vi "运维调试_采配水.vi"() -> ()   [LabVIEW 2016, in "PLC.lvlib"]
uses:
  PLC.lvlib
  <vilib>/Plasmionique/MB Master/MB_Master/MB_Master.lvclass
  <vilib>/Utility/miscctls.llb/LVPointTypeDef.ctl
  <vilib>/Plasmionique/MB Master/MB_Master_Serial/MB_Master_Serial.lvclass
  D:/Program Files (x86)/National Instruments/LabVIEW 2016/vi.lib/Plasmionique/MB Master/MB_Master/MB_Master.lvclass
  <vilib>/Utility/config.llb/Read Key (U32).vi
  <vilib>/Plasmionique/MB Master/MB Master.lvlib
  <vilib>/Utility/config.llb/NI_LVConfig.lvlib
panel:
  out "R22":i16
  in  "V8":bool
  out "R111":i16 caption="排液时间"
  out "通讯故障":bool
  out "R21":i16
  in  "V7":bool
  out "R20":i16
  in  "M1-2":bool
  in  "潜水泵工作模式":u16(ring) items=["泵1单泵单管路", "泵2单泵单管路", "双泵双管路"]
  out "X10":bool caption="废液报警"
  out "X9":bool caption="自来水报警"
  out "X8":bool caption="泵2过载报警"
  out "X7":bool caption="泵1过载报警"
  out "X6":bool caption="断电检测"
  out "X5":bool caption="开门检测"
  out "X4":bool caption="烟雾检测"
  out "X3":bool caption="漏水检测"
  out "X2":bool caption="进样检测"
  out "X1":bool
  out "X0":bool caption="采样池液位开关"
  out "Y12":bool caption="多参通电"
  out "R109":i16 caption="配水时间"
  out "集成报警信息":string
  out "R108":i16 caption="自来水报警"
  out "R107":i16 caption="采水池液位报警设置"
  out "R106":i16 caption="进样超时设置"
  out "R105":i16 caption="二级清洗时间"
  out "R104":i16 caption="一级清洗时间"
  out "R103":i16 caption="外部管路清洗时间"
  out "R102":i16 caption="静置沉淀时间"
  out "R101":i16 caption="内部管路润洗时间"
  out "R100":i16 caption="外部管路润洗时间"
  out "R2":i16
  out "R1":i16
  out "多列列表框":i32(listbox)
  out "R19":i16
  in  "V6":bool
  out "R18":i16
  in  "V5":bool
  out "R17":i16
  in  "V4":bool
  out "R16":i16
  in  "V3":bool
  out "R15":i16
  in  "V2":bool
  out "R14":i16
  in  "M2":bool
  out "R13":i16
  in  "V1":bool
  out "R12":i16
  in  "M1-1":bool
  in  "返回":bool
  in  "参数设置":bool
  in  "单步启动":bool
  in  "启动":bool
  in  "停止":bool
  # "S"
  # "S"
  # "S"
  # "S"
  # "S"
  # "S"
  # "S"
  # "S"
  # "S"
  # "S"
  # "S"
  # "单步计时："
  # "s"
  # "流程计时："
  # "s"
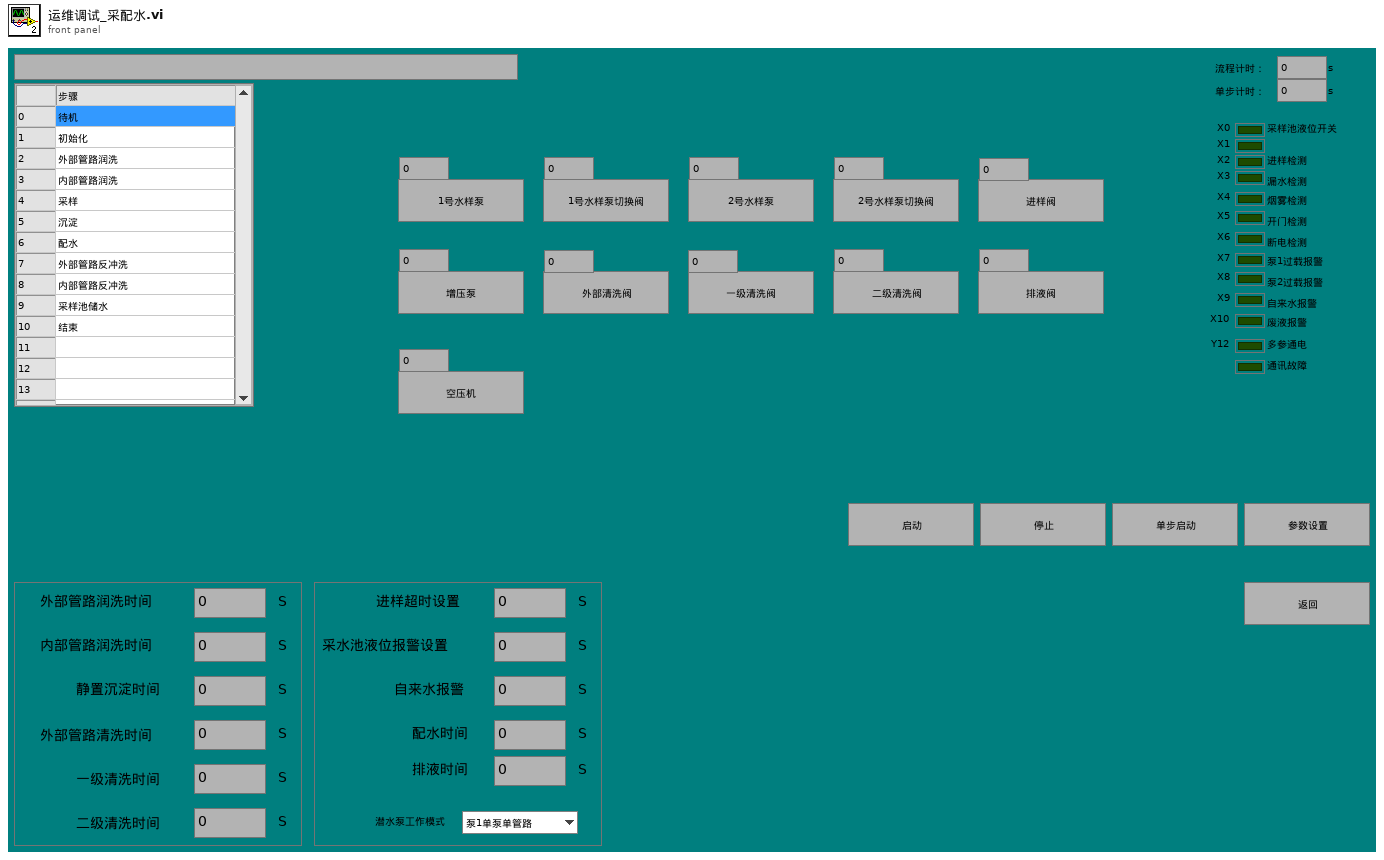
[diagram p1: front panel]
types:
  T1 = typedef "LVPointTypeDef.ctl" = cluster{"Horizontal":i16, "Vertical":i16}
  T2 = cluster{"时间标识":timestamp, "设备":string, "日志信息":string}
  T3 = cluster{"R0":i16, "R1":i16, "R2":i16, "R3":i16, "R4":i16, "R5":i16, "R6":i16, "R7":i16, "R8":i16, "R9":i16, "R10":i16, "R11":i16, "R12":i16, "R13":i16, "R14":i16, "R15":i16, "R16":i16, "R17":i16, "R18":i16, "R19":i16, "R20":i16, "R21":i16, "R22":i16}
  T4 = cluster{"coil values[0]":bool, "coil values[1]":bool, "coil values[2]":bool, "coil values[3]":bool, "coil values[4]":bool, "coil values[5]":bool, "coil values[6]":bool, "coil values[7]":bool, "coil values[8]":bool, "coil values[9]":bool, "coil values[10]":bool, "coil values[11]":bool, "coil values[12]":bool, "coil values[13]":bool, "coil values[14]":bool, "coil values[15]":bool}
  T5 = cluster{"seconds since 1Jan1904":timestamp, "table输入":string, string, "table输入":string}
  T6 = cluster{"时间标识":timestamp, "设备":string, "日志信息":string, "流程参数":string}
  T7 = cluster{"命令":string, cluster{"starting address":u16, "holding register value":u16}}
  T8 = cluster{"是否启用仪器":bool, "CODMn":cluster{"启动测量模式":cluster{"测量模式":enum16{"水样测量", "标样核查", "零点核查", "加标回收", "平行样", "校零", "校标"}}, "确定按钮":bool}, "采水模式":enum16{"使用采水泵", "不使用采水泵"}}
  T9 = enum16{"水样测量", "标样核查", "零点核查", "加标回收", "平行样", "校零", "校标"}
  T10 = cluster{"命令":string, "数据":cluster{"starting address":u16, "holding register value":u16}}
  T11 = cluster{"命令":string, "数据":cluster{"starting address":u16, "holding register values":u16[]}}
  T12 = cluster{"命令":string, "data":cluster{"starting address":u16, "coil values":bool[]}}
  T13 = enum32{"Bad", "Idle", "Run top level", "Running"}
  T14 = typedef "NI_LVConfig.lvlib/Config Data RefNum.ctl" = refnum<k1>
  T15 = cluster{"baud rate (bps)":u32, "stop bits":u16, "parity":u16, "flow control":u16, "timeout":u32, "retries":i32}
  T16 = cluster{"starting address":u16, "holding register values":u16[]}
  T17 = cluster{"starting address":u16, "holding register value":u16}
  T18 = cluster{"starting address":u16, "coil values":bool[]}
  T19 = cluster{"Registers[0]":u16, "Registers[1]":u16, "Registers[2]":u16, "Registers[3]":u16, "Registers[4]":u16, "Registers[5]":u16, "Registers[6]":u16, "Registers[7]":u16, "Registers[8]":u16, "Registers[9]":u16, "Registers[10]":u16, "Registers[11]":u16, "Registers[12]":u16, "Registers[13]":u16, "Registers[14]":u16, "Registers[15]":u16, "Registers[16]":u16, "Registers[17]":u16, "Registers[18]":u16, "Registers[19]":u16, "Registers[20]":u16, "Registers[21]":u16, "Registers[22]":u16}
  T20 = cluster{"Registers[0]":u16, "Registers[1]":u16, "Registers[2]":u16, "Registers[3]":u16, "Registers[4]":u16, "Registers[5]":u16}
  T21 = cluster{"Coils[0]":bool, "Coils[1]":bool, "Coils[2]":bool, "Coils[3]":bool, "Coils[4]":bool, "Coils[5]":bool, "Coils[6]":bool, "Coils[7]":bool, "Coils[8]":bool, "Coils[9]":bool, "Coils[10]":bool, "Coils[11]":bool, "Coils[12]":bool, "Coils[13]":bool, "Coils[14]":bool, "Coils[15]":bool}
  T22 = cluster{"Registers[0]":u16, "Registers[1]":u16, "Registers[2]":u16, "Registers[3]":u16, "Registers[4]":u16, "Registers[5]":u16, "Registers[6]":u16, "Registers[7]":u16, "Registers[8]":u16, "Registers[9]":u16, "Registers[10]":u16, "Registers[11]":u16, "Registers[12]":u16, "Registers[13]":u16, "Registers[14]":u16, "Registers[15]":u16, "Registers[16]":u16, "Registers[17]":u16, "Registers[18]":u16, "Registers[19]":u16}
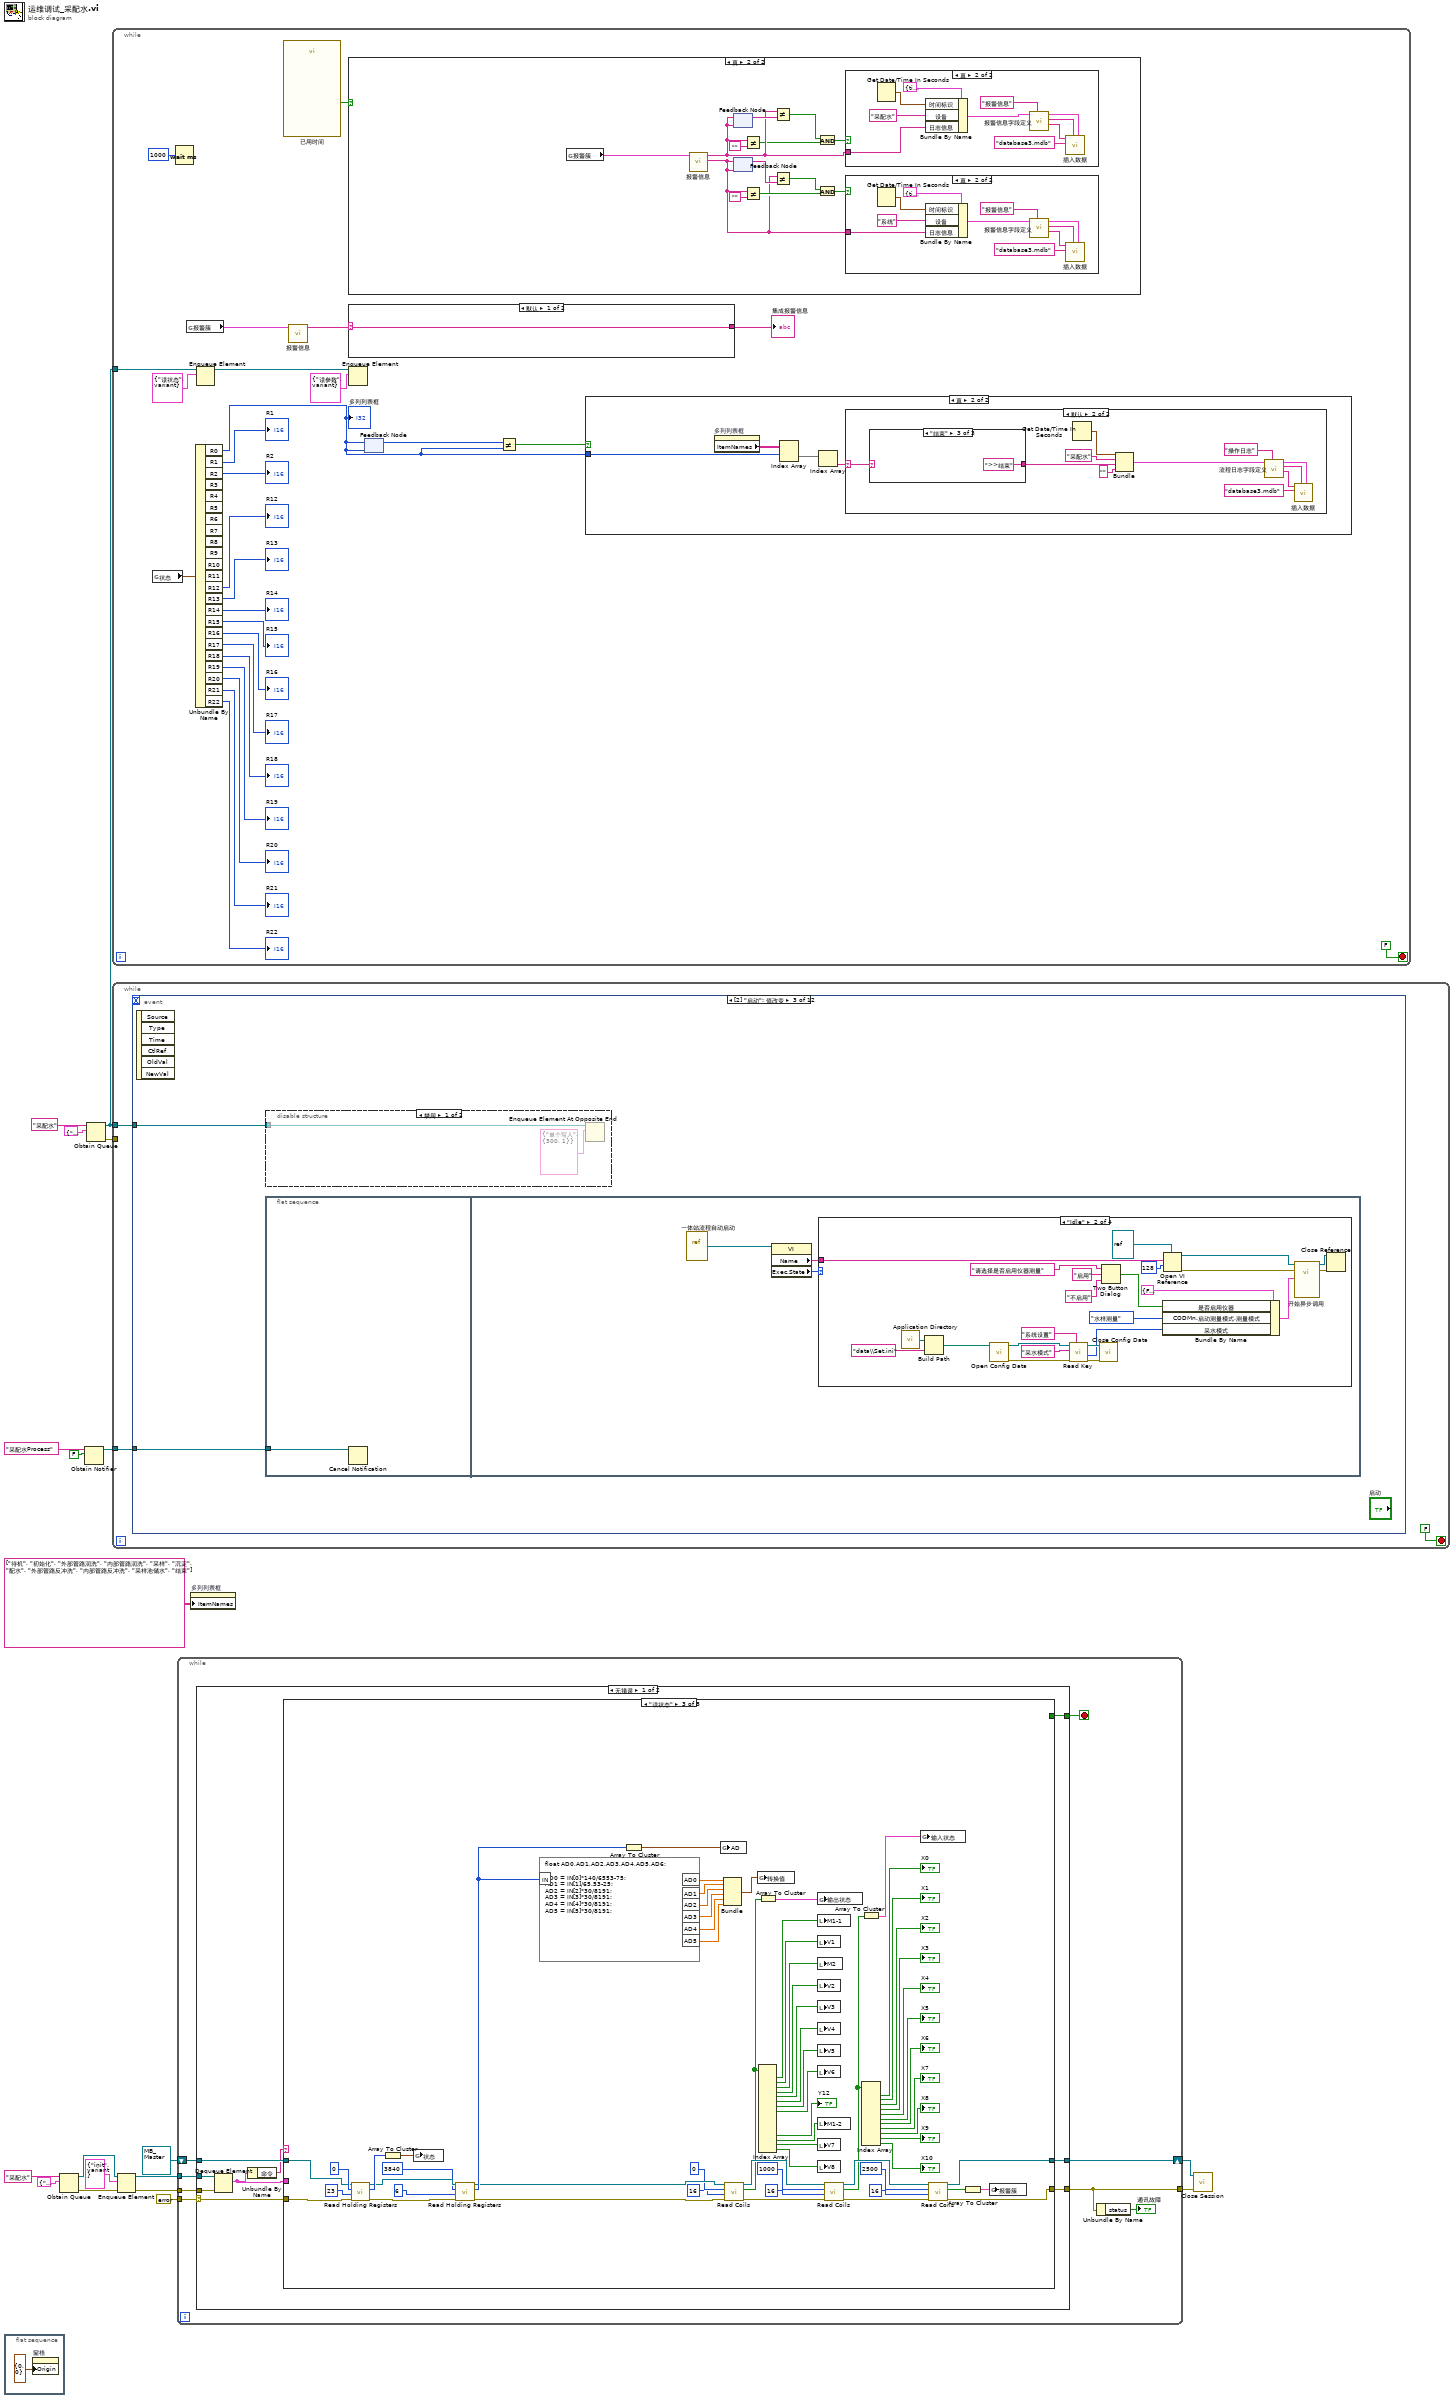
[diagram p0: block diagram]
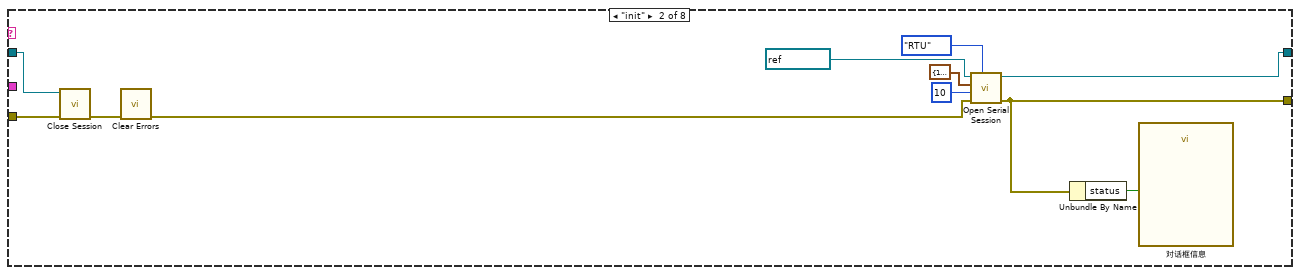
[diagram p3: hidden frame]
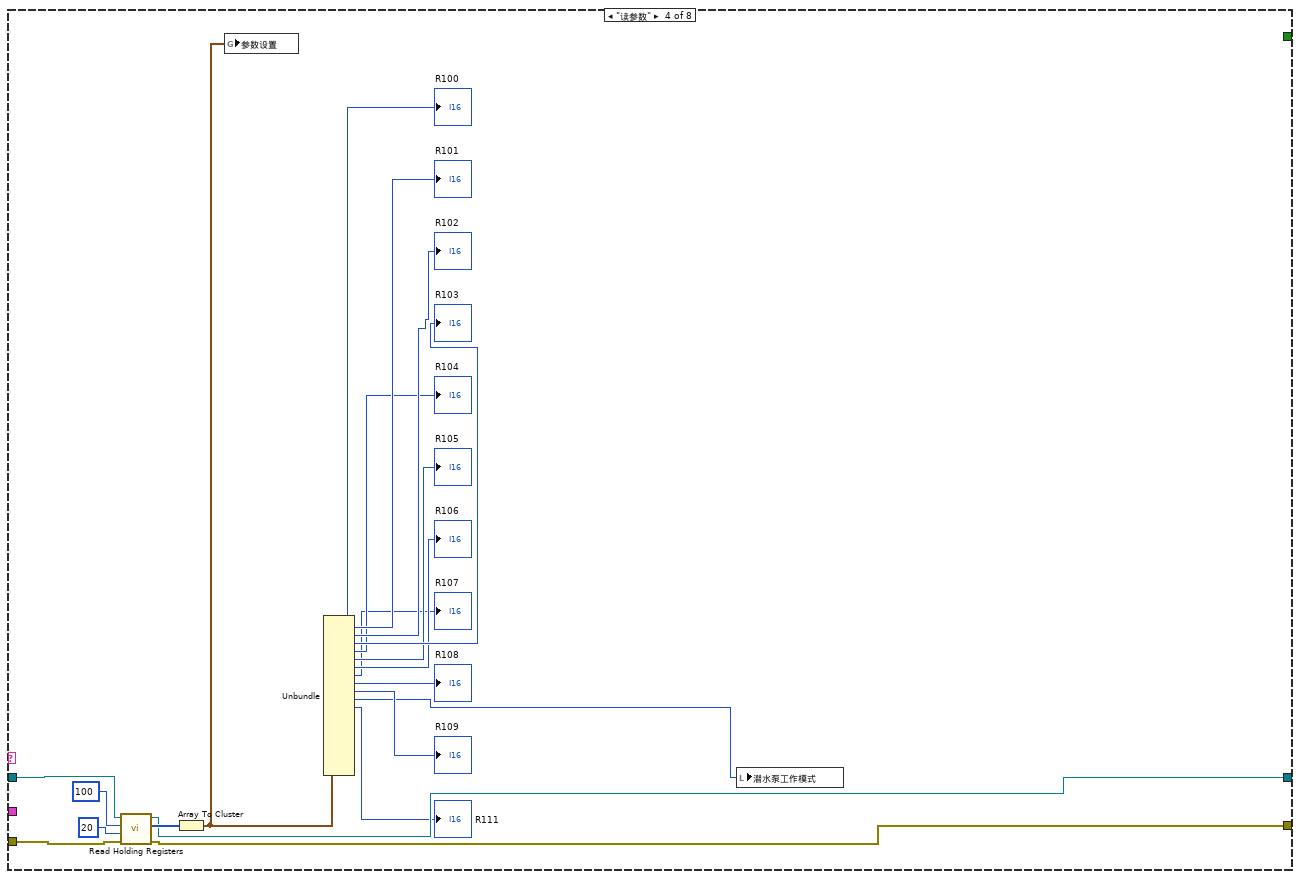
[diagram p4: hidden frame]
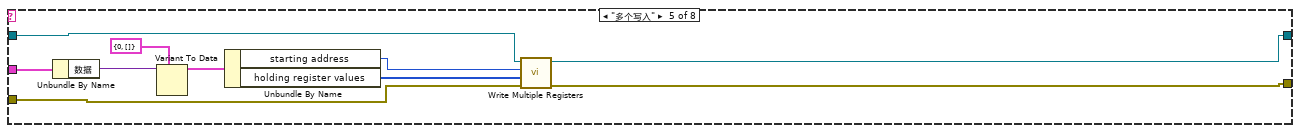
[diagram p5: hidden frame]
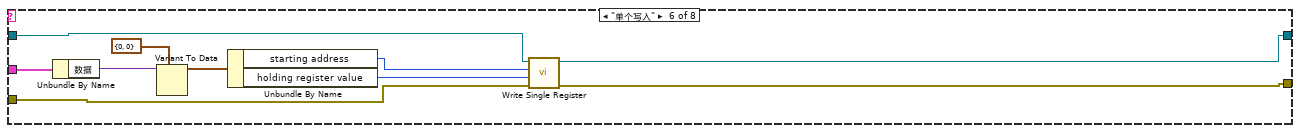
[diagram p6: hidden frame]
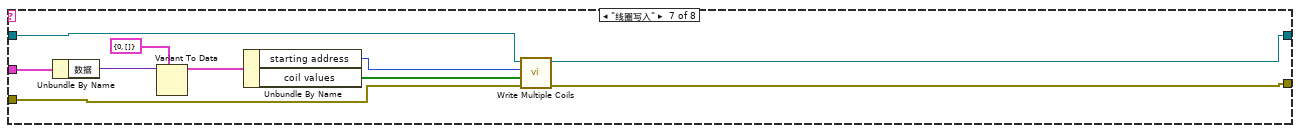
[diagram p7: hidden frame]
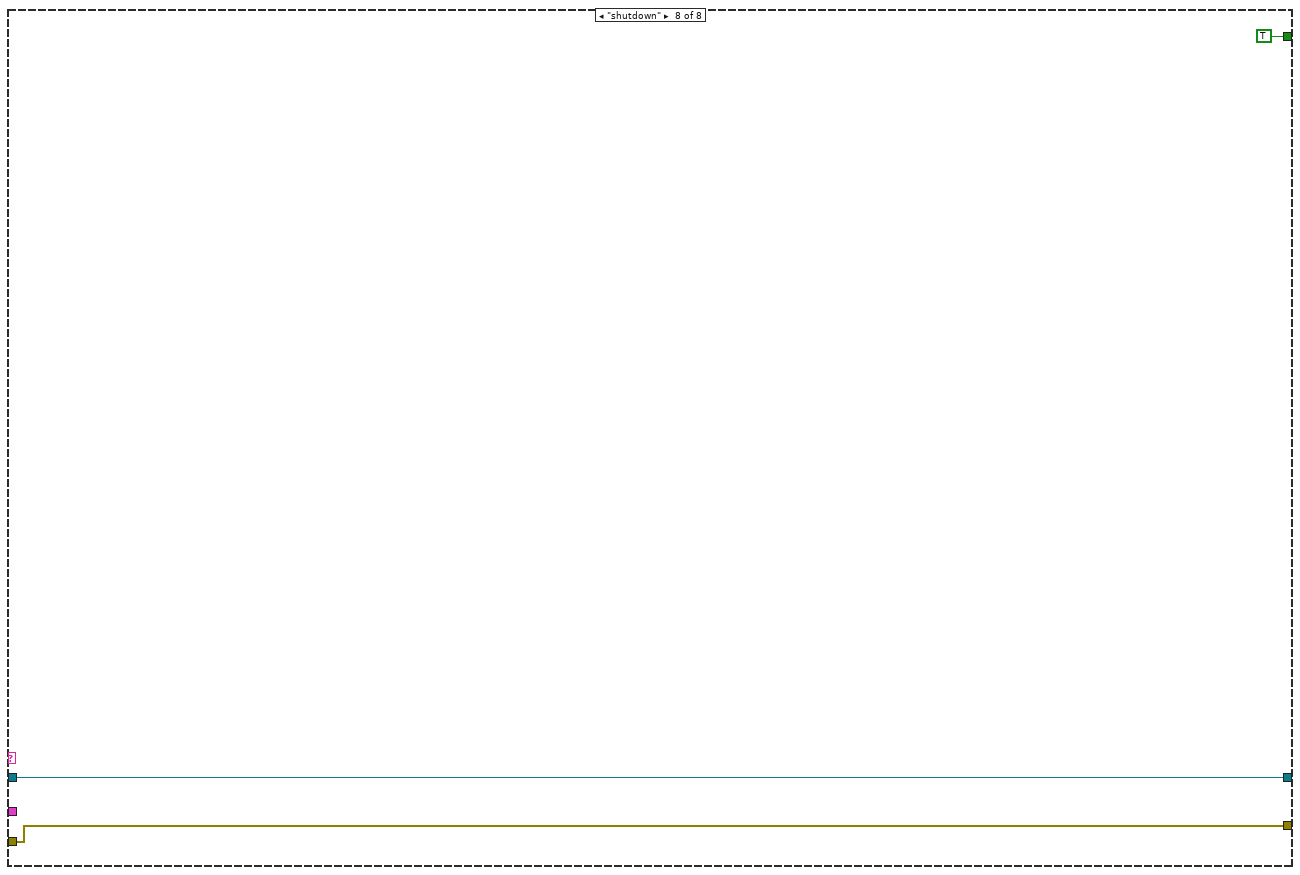
[diagram p8: hidden frame]
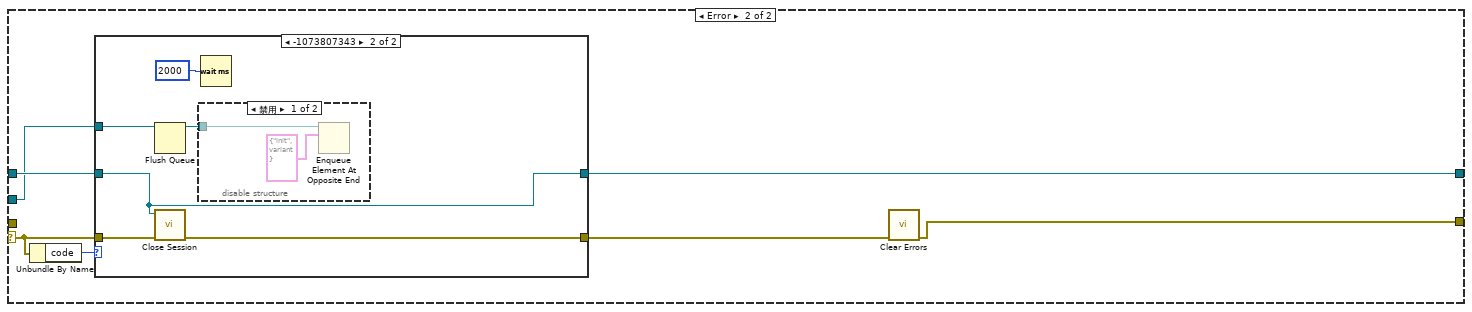
[diagram p9: hidden frame]
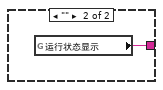
[diagram p15: hidden frame]
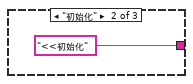
[diagram p19: hidden frame]
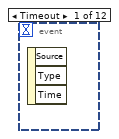
[diagram p20: hidden frame]
diagram:
  n1 = flat-sequence {
    frame #0 {
      n2 = property on="窗格" class="Pane"("Origin"=T1 {"Horizontal"=0, "Vertical"=0} ("原点")) -> ()  [unwired: 2 in, 2 out]
    }
  }
  n3 = Obtain Queue(name (unnamed)="采配水" ("名称（未命名）"), element data type=cluster{"命令":string, "数据":variant} {"命令"="", "数据"=variant}) -> (queue out=w9:refnum<queue>, error out=w8:errorcluster)  [unwired: 3 in, 1 out]
  n4 = Obtain Notifier(name (unnamed)="采配水Process" ("名称（未命名）"), notification data type=FALSE) -> (notifier out=w12:refnum<notifier>)  [unwired: 2 in, 2 out]
  n5 = Obtain Queue(name (unnamed)="采配水" ("名称（未命名）"), element data type=cluster{"命令":string, "数据":variant} {"命令"="", "数据"=variant}) -> (queue out=w16:refnum<queue>, error out=w17:errorcluster)  [unwired: 3 in, 1 out]
  n6 = while {
    tunnel: w16 -> [w46]
    stop <- FALSE stop-if-true
    n7 = global read "采配水全局变量.vi" "状态"() -> (w44:T3)
    n8 = Wait (ms)(milliseconds to wait=u32 1000 ("等待时间（毫秒）")) -> ()  [unwired: 1 out]
    n9 = global read "采配水全局变量.vi" "报警簇"() -> (w32:T4)
    n10 = Unbundle By Name(w44) -> ("R0"=w25:i16, "R1"=→"R1":i16, "R2"=→"R2":i16, "R12"=→"R12":i16, "R13"=→"R13":i16, "R14"=→"R14":i16, "R15"=→"R15":i16, "R16"=→"R16":i16, "R17"=→"R17":i16, "R18"=→"R18":i16, "R19"=→"R19":i16, "R20"=→"R20":i16, "R21"=→"R21":i16, "R22"=→"R22":i16)  [unwired: 9 out]
    "多列列表框" <- w25
    n11 = Enqueue Element(queue=w46, element=cluster{"命令":string, "数据":variant} {"命令"="读状态", "数据"=variant} ("元素")) -> (queue out=w27:refnum<queue>)  [unwired: 2 in, 2 out]
    n12 = call "已用时间"() -> ("Time has Elapsed"=w30:bool)  [unwired: 12 in, 7 out]
    n13 = call "报警信息.vi"("报警簇"=w32) -> ("采配水报警信息"=w24:string)  [unwired: 9 in, 1 out]
    n14 = case shown="真" w30 {
      frame False {
      }
      frame True {
        n15 = global read "采配水全局变量.vi" "报警簇"() -> (w60:T4)
        n16 = call "报警信息.vi"("报警簇"=w60) -> ("系统报警信息"=w49:string, "采配水报警信息"=w56:string)  [unwired: 9 in]
        n17 = feedback #1(w56) -> (w59:string)
        n18 = feedback-in #1(w56) -> ()
        n19 = feedback #2(w49) -> (w50:string)
        n20 = feedback-in #2(w49) -> ()
        n21 = Not Equal?(x=w56, y="") -> (x != y?=w54:bool)
        n22 = Not Equal?(x=w49, y="") -> (x != y?=w53:bool)
        n23 = Not Equal?(x=w56, y=w59) -> (x != y?=w58:bool)
        n24 = Not Equal?(x=w49, y=w50) -> (x != y?=w51:bool)
        n25 = And(x=w58, y=w54) -> (x .and. y?=w57:bool)
        n26 = And(x=w51, y=w53) -> (x .and. y?=w48:bool)
        n27 = case shown="真" w57 {
          tunnel: w56 -> [_ w71]
          frame False {
          }
          frame True {
            n28 = Get Date/Time In Seconds() -> (seconds since 1Jan1904=w73:timestamp)
            n29 = Bundle By Name(cluster=T2 {"时间标识"=timestamp(0 s since 1904-01-01), "设备"="", "日志信息"=""} ("data in"), "时间标识"=w73, "设备"="采配水", "日志信息"=w71) -> (w74:T2)
            n30 = call "报警信息字段定义.vi"("table输入"="报警信息", "data in"=w74) -> ("table输出"=w78:string, "columns"=w79:string[], "data out"=w80:T2)  [unwired: 7 in]
            n31 = call "插入数据.vi"("data"=w80, "columns"=w79, "database"="database3.mdb", "table"=w78) -> ()  [unwired: 7 in, 1 out]
          }
        }
        n32 = case shown="真" w48 {
          tunnel: w49 -> [_ w61]
          frame False {
          }
          frame True {
            n33 = Get Date/Time In Seconds() -> (seconds since 1Jan1904=w63:timestamp)
            n34 = Bundle By Name(cluster=T2 {"时间标识"=timestamp(0 s since 1904-01-01), "设备"="", "日志信息"=""} ("data in"), "时间标识"=w63, "设备"="系统", "日志信息"=w61) -> (w64:T2)
            n35 = call "报警信息字段定义.vi"("table输入"="报警信息", "data in"=w64) -> ("table输出"=w68:string, "columns"=w69:string[], "data out"=w70:T2)  [unwired: 7 in]
            n36 = call "插入数据.vi"("data"=w70, "columns"=w69, "database"="database3.mdb", "table"=w68) -> ()  [unwired: 7 in, 1 out]
          }
        }
      }
    }
    n37 = case shown="默认" w24 {
      selector: w24 -> [w81 _]
      tunnel: [w81 w82] -> w31
      frame Default {
      }
      frame "" {
        n38 = global read "采配水全局变量.vi" "运行状态显示"() -> (w82:string)
      }
    }
    "集成报警信息" <- w31
    n39 = Enqueue Element(queue=w27, element=cluster{"命令":string, "数据":variant} {"命令"="读参数", "数据"=variant} ("元素")) -> ()  [unwired: 2 in, 3 out]
    n40 = feedback-in #3(w25) -> ()
    n41 = feedback #3(w25) -> (w26:i16)
    n42 = Not Equal?(x=w26, y=w25) -> (x != y?=w33:bool)
    n43 = case shown="真" w33 {
      tunnel: w25 -> [_ w85]
      frame False {
      }
      frame True {
        n44 = property on="多列列表框" class="MCListbox (严格)"() -> ("ItemNames"=w86:string[][])  [unwired: 2 in, 2 out]
        n45 = Index Array(array=w86, index (row)=w85) -> (element=w84:string[])  [unwired: 1 in]
        n46 = Index Array(array=w84) -> (element=w83:string)  [unwired: 1 in]
        n47 = case shown="默认" w83 {
          selector: w83 -> [_ w88]
          frame "待机" {
          }
          frame Default {
            n48 = case shown="\"结束\"" w88 {
              selector: w88 -> [w98 _ _]
              tunnel: [w98 "<<初始化" ">>结束"] -> w87
              frame Default {
              }
              frame "初始化" {
              }
              frame "结束" {
              }
            }
            n49 = Get Date/Time In Seconds() -> (seconds since 1Jan1904=w92:timestamp)
            n50 = Bundle("seconds since 1Jan1904"=w92, "table输入"="采配水", w87, "table输入"="") -> (w90:T5)  [unwired: 1 in]
            n51 = call "流程日志字段定义.vi"("table输入"="操作日志", "data in"=w90) -> ("table输出"=w95:string, "columns"=w96:string[], "data out"=w97:T6)  [unwired: 7 in]
            n52 = call "插入数据.vi"("data"=w97, "columns"=w96, "database"="database3.mdb", "table"=w95) -> ()  [unwired: 7 in, 1 out]
          }
        }
      }
    }
  }
  n53 = while {
    tunnel: w16 -> [w102]
    tunnel: w17 -> [_]
    tunnel: w12 -> [w101]
    stop <- FALSE stop-if-true
    n54 = event shown="[2] \"启动\": 值改变" {
      selector: _ -> [_ _ _ _ _ _ _ _ _ _ _ _]
      dyn-events: _ -> [_ _ _ _ _ _ _ _ _ _ _ _]
      timeout: _ -> [_ _ _ _ _ _ _ _ _ _ _ _]
      tunnel: w102 -> [_ w106 w109 w144 w161 _ _ _ w179 w181 w186 w191]
      tunnel: w101 -> [_ w105 w108 _ _ _ _ _ _ _ _ _]
      event Timeout {
        n55 = event-data() -> ()  [unwired: 1 in, 3 out]
      }
      event "停止": Value Change {
        n56 = event-data() -> ()  [unwired: 1 in, 6 out]
        n57 = Send Notification(notification=TRUE ("通知"), notifier=w105) -> ()  [unwired: 1 in, 2 out]
        n58 = Enqueue Element At Opposite End(queue=w106, element=T7 {"命令"="单个写入", {"starting address"=300, "holding register value"=2}} ("元素")) -> ()  [unwired: 2 in, 3 out]
      }
      event "启动": Value Change {
        n59 = event-data() -> ()  [unwired: 1 in, 6 out]
        n60 = disable-structure shown="禁用" {
          disable-tunnel: w109 -> [w140 _]
          frame Disabled {
            n61 = Enqueue Element At Opposite End(queue=w140, element=T7 {"命令"="单个写入", {"starting address"=300, "holding register value"=1}} ("元素")) -> ()  [unwired: 2 in, 3 out]
          }
          frame Enabled {
          }
        }
        n62 = flat-sequence {
          tunnel: w108 -> [w110]
          frame #0 {
            n63 = Cancel Notification(0:w110) -> ()  [unwired: 1 in, 3 out]
          }
          frame #1 {
            n64 = vi-ref "一体站流程自动启动.vi"() -> (w113:refnum<vi>)
            n65 = property class="VI"(reference=w113) -> ("Name"=w112:string, "Exec.State"=w111:T13)  [unwired: 1 in, 2 out]
            n66 = case shown="\"Idle\"" w111 {
              tunnel: w112 -> [_ w137 _ _]
              frame "Bad", Default {
              }
              frame "Idle" {
                n67 = call <vilib>:"Application Directory.vi"() -> ("Application Directory"=w121:path)
                n68 = Build Path(base path=w121, name or relative path="data\\Set.ini" ("名称或相对路径")) -> (appended path=w119:path)
                n69 = call <vilib>:"Open Config Data.vi"("configuration file path"=w119) -> ("error out"=w122:errorcluster, "refnum"=w123:T14)  [unwired: 8 in, 1 out]
                n70 = call-poly <vilib>:"Read Key.vi"("section"="系统设置", "error in (no error)"=w122, "key"="采水模式", "refnum"=w123) -> ("error out"=w117:errorcluster, "value"=w114:u32, "refnum out"=w118:T14)  [unwired: 4 in, 1 out]
                n71 = call <vilib>:"Close Config Data.vi"("error in (no error)"=w117, "refnum"=w118) -> ()  [unwired: 8 in, 2 out]
                n72 = Two Button Dialog(message="请选择是否启用仪器测量" ("消息"), 1:"不启用" ("F按钮名称（“取消”）"), 2:"启用" ("T按钮名称（“确定”）")) -> (T button?=w127:bool)
                n73 = Bundle By Name(cluster=T8 {"是否启用仪器"=FALSE, "CODMn"={"启动测量模式"={"测量模式"=enum."水样测量"}, "确定按钮"=FALSE}, "采水模式"=enum."使用采水泵"} ("参数"), "是否启用仪器"=w127, "CODMn.启动测量模式.测量模式"=T9."水样测量", "采水模式"=w114) -> (w124:T8)
                n74 = Open VI Reference(type specifier VI Refnum (for type only)=refnum<vi> refnum, vi path=w137, options=128 ("选项")) -> (vi reference=w135:refnum<vi>, error out=w132:errorcluster)  [unwired: 3 in]
                n75 = call-by-ref "开始异步调用"(reference=w135, error in=w132, "参数"=w124) -> (reference out=w133:refnum<vi>, error out=w131:errorcluster)  [unwired: 11 in]
                n76 = Close Reference(reference=w133, error in (no error)=w131) -> ()  [unwired: 1 out]
              }
              frame "Run top level" {
              }
              frame "Running" {
                n77 = One Button Dialog(message="流程已经运行,无须重复启动" ("消息")) -> ()  [unwired: 1 in, 1 out]
              }
            }
          }
        }
      }
      event "单步启动": Value Change {
        n78 = event-data() -> ()  [unwired: 1 in, 6 out]
        n79 = call "单步启动对话框.vi"() -> ("单步启动步骤输出"=w141:u16)  [unwired: 11 in]
        n80 = Bundle By Name(cluster=T10 {"命令"="单个写入", "数据"={"starting address"=301, "holding register value"=0}} ("元素"), "数据.holding register value"=w141) -> (w142:T10)
        n81 = Enqueue Element At Opposite End(queue=w144, element=w142) -> ()  [unwired: 2 in, 3 out]
      }
      event "R100", "R101", "R102", "R103", "R104", "R105", "R106", "R107", "R108", "R109", "潜水泵工作模式", "R111": Value Change {
        n82 = event-data() -> ()  [unwired: 1 in, 6 out]
        n83 = local read "R100"() -> (w156:i16)
        n84 = local read "R101"() -> (w155:i16)
        n85 = local read "R102"() -> (w154:i16)
        n86 = local read "R103"() -> (w153:i16)
        n87 = local read "R104"() -> (w152:i16)
        n88 = local read "R105"() -> (w151:i16)
        n89 = local read "R106"() -> (w150:i16)
        n90 = local read "R107"() -> (w149:i16)
        n91 = local read "R108"() -> (w148:i16)
        n92 = local read "R109"() -> (w147:i16)
        n93 = local read "R111"() -> (w145:i16)
        n94 = Build Array(w156, w155, w154, w153, w152, w151, w150, w149, w148, w147, "潜水泵工作模式", w145) -> (w157:u16[])
        n95 = Bundle By Name(cluster=T11 {"命令"="多个写入", "数据"={"starting address"=0, "holding register values"=[]}} ("元素"), "数据.starting address"=u16 100, "数据.holding register values"=w157) -> (w158:T11)
        n96 = Enqueue Element At Opposite End(queue=w161, element=w158) -> ()  [unwired: 2 in, 3 out]
      }
      event "R100", "R101", "R102", "R103", "R104", "R105", "R106", "R107", "R108", "R109", "R111": Mouse Down {
        n97 = event-data() -> ("CtlRef"=w165:refnum<vi>)  [unwired: 1 in, 7 out]
        n98 = property class="DigNum (严格)"(reference=w165) -> (reference out=w163:refnum<vi>, "Value"=w164:i16)  [unwired: 1 in, 1 out]
        n99 = call "数字键盘.vi"("OldNumber"=w164) -> ("NewNumber"=w162:sgl)
        n100 = property class="DigNum (严格)"(reference=w163, "Val(Sgnl)"=w162) -> ()  [unwired: 1 in, 2 out]
      }
      event "参数设置": Value Change {
        n101 = event-data() -> ()  [unwired: 1 in, 6 out]
        n102 = property on="窗格" class="Pane"("Origin"=T1 {"Horizontal"=0, "Vertical"=528} ("原点")) -> ()  [unwired: 2 in, 2 out]
      }
      event "返回": Value Change {
        n103 = event-data() -> ()  [unwired: 1 in, 6 out]
        n104 = property on="窗格" class="Pane"("Origin"=T1 {"Horizontal"=0, "Vertical"=0} ("原点")) -> ()  [unwired: 2 in, 2 out]
      }
      event "M1-1", "V1", "M2", "V2", "V3", "V4", "V5", "V6": Value Change {
        n105 = event-data() -> ()  [unwired: 1 in, 6 out]
        n106 = Build Array("M1-1", "V1", "M2", "V2", "V3", "V4", "V5", "V6") -> (w168:bool[])
        n107 = Bundle By Name(cluster=T12 {"命令"="线圈写入", "data"={"starting address"=2400, "coil values"=[]}} ("元素"), "data.coil values"=w168) -> (w169:T12)
        n108 = Enqueue Element(queue=w179, element=w169) -> ()  [unwired: 2 in, 3 out]
      }
      event "M1-2": Value Change {
        n109 = event-data() -> ()  [unwired: 1 in, 6 out]
        n110 = Build Array("M1-2") -> (w182:bool[])
        n111 = Bundle By Name(cluster=T12 {"命令"="线圈写入", "data"={"starting address"=2413, "coil values"=[]}} ("元素"), "data.coil values"=w182) -> (w183:T12)
        n112 = Enqueue Element(queue=w181, element=w183) -> ()  [unwired: 2 in, 3 out]
      }
      event "V7": Value Change {
        n113 = event-data() -> ()  [unwired: 1 in, 6 out]
        n114 = Build Array("V7") -> (w187:bool[])
        n115 = Bundle By Name(cluster=T12 {"命令"="线圈写入", "data"={"starting address"=2414, "coil values"=[]}} ("元素"), "data.coil values"=w187) -> (w188:T12)
        n116 = Enqueue Element(queue=w186, element=w188) -> ()  [unwired: 2 in, 3 out]
      }
      event "V8": Value Change {
        n117 = event-data() -> ()  [unwired: 1 in, 6 out]
        n118 = Build Array("V8") -> (w192:bool[])
        n119 = Bundle By Name(cluster=T12 {"命令"="线圈写入", "data"={"starting address"=2415, "coil values"=[]}} ("元素"), "data.coil values"=w192) -> (w193:T12)
        n120 = Enqueue Element(queue=w191, element=w193) -> ()  [unwired: 2 in, 3 out]
      }
    }
  }
  n121 = Enqueue Element(queue=w9, element=cluster{"命令":string, "数据":variant} {"命令"="init", "数据"=variant} ("元素"), error in (no error)=w8) -> (queue out=w4:refnum<queue>, error out=w6:errorcluster)  [unwired: 1 in, 1 out]
  n122 = while {
    tunnel: w4 -> [w199]
    tunnel: w6 -> [w198]
    shift-right: [w202] -> w1
    shift-left: refnum<class "MB_Master.lvclass"> refnum ("MB session in") -> [w201]
    tunnel: errorcluster {"status"=FALSE, "code"=0, "source"=""} ("error out") -> [w200]
    tunnel: [w196] -> w2
    stop <- w197 stop-if-true
    n123 = case shown="无错误" w200 {
      selector: w200 -> [w208 w344]
      tunnel: [w211 w343] -> w202
      tunnel: w201 -> [w210 w345]
      tunnel: [w209 w341] -> w196
      tunnel: w199 -> [w205 w340]
      tunnel: w198 -> [w204 _]
      tunnel: [w206 _] -> w197
      frame No Error {
        n124 = Dequeue Element(queue=w205, error in (no error)=w204) -> (element=w203:cluster{"命令":string, "数据":variant})  [unwired: 1 in, 3 out]
        n125 = Unbundle By Name(w203) -> ("命令"=w207:string)
        n126 = case shown="\"读状态\"" w207 {
          tunnel: [w213 w217 w251 w301 w313 w323 w333 w338] -> w211
          tunnel: w210 -> [w213 w221 w271 w306 w316 w326 w336 w338]
          tunnel: [w212 w219 w250 w300 w314 w324 w334 w337] -> w209
          tunnel: w208 -> [w212 w223 w274 w305 w315 w325 w335 w337]
          tunnel: [_ _ _ _ _ _ _ TRUE] -> w206
          tunnel: w203 -> [_ _ _ _ w312 w322 w332 _]
          frame "idle", Default {
          }
          frame "init" {
            n127 = call-dynamic "Close Session.vi"("error in (no error)"=w223, "MB session in"=w221) -> ("error out"=w222:errorcluster)  [unwired: 9 in]
            n128 = call <vilib>:"Clear Errors.vi"("error in (no error)"=w222) -> ("error out"=w220:errorcluster)  [unwired: 5 in, 1 out]
            n129 = call <vilib>:"Open Serial Session.vi"("Mode (RTU)"=enum16{"RTU", "ASCII"}."RTU", "Error in"=w220, "Slave ID"=u8 10, "Serial Config"=T15 {"baud rate (bps)"=115200, "stop bits"=10, "parity"=0, "flow control"=0, "timeout"=100, "retries"=1}, "VISA Resource"=refnum<visa-resource-name> "COM2" ("VISA resource name")) -> ("Error out"=w219:errorcluster, "MB_Serial session"=w217:refnum<class "MB_Master_Serial.lvclass">)  [unwired: 5 in]
            n130 = Unbundle By Name(w219) -> ("status"=w224:bool)
            n131 = call "对话框信息"("Enable"=w224) -> ()  [unwired: 9 in, 2 out]
          }
          frame "读状态" {
            n132 = call <vilib>:"Read Holding Registers.vi"("error in (no error)"=w274, "quantity"=u16 23 ("number of holding registers"), "starting address"=u16 0, "MB session in"=w271) -> ("error out"=w267:errorcluster, "Registers"=w270:u16[], "MB session out"=w269:refnum<class "MB_Master.lvclass">)  [unwired: 5 in]
            n133 = Array To Cluster(array=w270) -> (cluster=w276:T19)
            n134 = global write "采配水全局变量.vi" "状态"(w276) -> ()
            n135 = call <vilib>:"Read Holding Registers.vi"("error in (no error)"=w267, "quantity"=u16 6 ("number of holding registers"), "starting address"=u16 3840, "MB session in"=w269) -> ("error out"=w263:errorcluster, "Registers"=w268:u16[], "MB session out"=w264:refnum<class "MB_Master.lvclass">)  [unwired: 5 in]
            n136 = formula code="float AD0,AD1,AD2,AD3,AD4,AD5,AD6;\n\nAD0 = IN[0]*140/6553-75;\nAD1 = IN[1]/65.53-25;\nAD2 = IN[2]*30/8191;\nAD3 = IN[3]*30/8191;\nAD4 = IN[4]*30/8191;\nAD5 = IN[5]*30/8191;"("IN"=w268) -> ("AD0"=w282:dbl, "AD1"=w281:dbl, "AD2"=w280:dbl, "AD3"=w279:dbl, "AD4"=w278:dbl, "AD5"=w277:dbl)
            n137 = Array To Cluster(array=w268) -> (cluster=w284:T20)
            n138 = global write "采配水全局变量.vi" "AD"(w284) -> ()
            n139 = Bundle(w282, w281, w280, w279, w278, w277) -> (w283:cluster{dbl, dbl, dbl, dbl, dbl, dbl})  [unwired: 1 in]
            n140 = call <vilib>:"Read Coils.vi"("error in (no error)"=w263, "quantity"=u16 16 ("number of coils"), "starting address"=u16 0, "MB session in"=w264) -> ("error out"=w259:errorcluster, "Coils"=w240:bool[], "MB session out"=w260:refnum<class "MB_Master.lvclass">)  [unwired: 5 in]
            n141 = global write "采配水全局变量.vi" "转换值"(w283) -> ()
            n142 = Index Array(array=w240) -> (element #1=w235:bool, element #2=w234:bool, element #3=w233:bool, element #4=w232:bool, element #5=w231:bool, element #6=w230:bool, element #7=w229:bool, element #8=w228:bool, element #13=→"Y12":bool, element #14=w227:bool, element #15=w226:bool, element #16=w225:bool)  [unwired: 16 in, 4 out]
            n143 = Array To Cluster(array=w240) -> (cluster=w285:T21)
            n144 = global write "采配水全局变量.vi" "输出状态"(w285) -> ()
            n145 = local write "M1-1"(w235) -> ()
            n146 = local write "V1"(w234) -> ()
            n147 = local write "M2"(w233) -> ()
            n148 = local write "V2"(w232) -> ()
            n149 = local write "V3"(w231) -> ()
            n150 = local write "V4"(w230) -> ()
            n151 = local write "V5"(w229) -> ()
            n152 = local write "V6"(w228) -> ()
            n153 = local write "M1-2"(w227) -> ()
            n154 = local write "V7"(w226) -> ()
            n155 = local write "V8"(w225) -> ()
            n156 = call <vilib>:"Read Coils.vi"("error in (no error)"=w259, "quantity"=u16 16 ("number of coils"), "starting address"=u16 1000, "MB session in"=w260) -> ("error out"=w255:errorcluster, "Coils"=w249:bool[], "MB session out"=w256:refnum<class "MB_Master.lvclass">)  [unwired: 5 in]
            n157 = Index Array(array=w249) -> (element #1=→"X0":bool, element #2=→"X1":bool, element #3=→"X2":bool, element #4=→"X3":bool, element #5=→"X4":bool, element #6=→"X5":bool, element #7=→"X6":bool, element #8=→"X7":bool, element #9=→"X8":bool, element #10=→"X9":bool, element #11=→"X10":bool)  [unwired: 11 in]
            n158 = Array To Cluster(array=w249) -> (cluster=w286:T21)
            n159 = global write "采配水全局变量.vi" "输入状态"(w286) -> ()
            n160 = call <vilib>:"Read Coils.vi"("error in (no error)"=w255, "quantity"=u16 16 ("number of coils"), "starting address"=u16 2500, "MB session in"=w256) -> ("error out"=w250:errorcluster, "Coils"=w252:bool[], "MB session out"=w251:refnum<class "MB_Master.lvclass">)  [unwired: 5 in]
            n161 = Array To Cluster(array=w252) -> (cluster=w275:T21)
            n162 = global write "采配水全局变量.vi" "报警簇"(w275) -> ()
          }
          frame "读参数" {
            n163 = call <vilib>:"Read Holding Registers.vi"("error in (no error)"=w305, "quantity"=u16 20 ("number of holding registers"), "starting address"=u16 100, "MB session in"=w306) -> ("error out"=w300:errorcluster, "Registers"=w302:u16[], "MB session out"=w301:refnum<class "MB_Master.lvclass">)  [unwired: 5 in]
            n164 = Array To Cluster(array=w302) -> (cluster=w289:T22)
            n165 = global write "采配水全局变量.vi" "参数设置"(w289) -> ()
            n166 = Unbundle(w289) -> ("Registers[0]"=→"R100":u16, "Registers[1]"=→"R101":u16, "Registers[2]"=→"R102":u16, "Registers[3]"=→"R103":u16, "Registers[4]"=→"R104":u16, "Registers[5]"=→"R105":u16, "Registers[6]"=→"R106":u16, "Registers[7]"=→"R107":u16, "Registers[8]"=→"R108":u16, "Registers[9]"=→"R109":u16, "Registers[10]"=w288:u16, "Registers[11]"=→"R111":u16)  [unwired: 8 out]
            n167 = local write "潜水泵工作模式"(w288) -> ()
          }
          frame "多个写入" {
            n168 = Unbundle By Name(w312) -> ("数据"=w311:variant)
            n169 = Variant To Data(type=T16 {"starting address"=0, "holding register values"=[]}, Variant=w311) -> (data=w309:T16)  [unwired: 1 in, 1 out]
            n170 = Unbundle By Name(w309) -> ("starting address"=w308:u16, "holding register values"=w307:u16[])
            n171 = call <vilib>:"Write Multiple Registers.vi"("error in (no error)"=w315, "values"=w307, "starting address"=w308, "MB session in"=w316) -> ("error out"=w314:errorcluster, "MB session out"=w313:refnum<class "MB_Master.lvclass">)  [unwired: 6 in]
          }
          frame "单个写入" {
            n172 = Unbundle By Name(w322) -> ("数据"=w321:variant)
            n173 = Variant To Data(type=T17 {"starting address"=0, "holding register value"=0}, Variant=w321) -> (data=w319:T17)  [unwired: 1 in, 1 out]
            n174 = Unbundle By Name(w319) -> ("starting address"=w318:u16, "holding register value"=w317:u16)
            n175 = call <vilib>:"Write Single Register.vi"("error in (no error)"=w325, "value"=w317, "address"=w318, "MB session in"=w326) -> ("error out"=w324:errorcluster, "MB session out"=w323:refnum<class "MB_Master.lvclass">)  [unwired: 6 in]
          }
          frame "线圈写入" {
            n176 = Unbundle By Name(w332) -> ("数据"=w331:variant)
            n177 = Variant To Data(type=T18 {"starting address"=0, "coil values"=[]}, Variant=w331) -> (data=w329:T18)  [unwired: 1 in, 1 out]
            n178 = Unbundle By Name(w329) -> ("starting address"=w328:u16, "coil values"=w327:bool[])
            n179 = call <vilib>:"Write Multiple Coils.vi"("error in (no error)"=w335, "values"=w327, "starting address"=w328, "MB session in"=w336) -> ("error out"=w334:errorcluster, "MB session out"=w333:refnum<class "MB_Master.lvclass">)  [unwired: 6 in]
          }
          frame "shutdown" {
          }
        }
      }
      frame Error {
        n180 = Unbundle By Name(w344) -> ("code"=w346:i32)
        n181 = case shown="-1073807343" w346 {
          tunnel: w345 -> [w348 w352]
          tunnel: w344 -> [w347 w354]
          tunnel: [w347 w353] -> w342
          tunnel: [w348 w352] -> w343
          tunnel: w340 -> [_ w351]
          frame Default {
          }
          frame -1073807343 {
            n182 = Flush Queue(queue=w351) -> (queue out=w350:refnum<queue>)  [unwired: 1 in, 2 out]
            n183 = call-dynamic "Close Session.vi"("error in (no error)"=w354, "MB session in"=w352) -> ("error out"=w353:errorcluster)  [unwired: 9 in]
            n184 = disable-structure shown="禁用" {
              disable-tunnel: w350 -> [w355 _]
              frame Disabled {
                n185 = Enqueue Element At Opposite End(queue=w355, element=cluster{"命令":string, "数据":variant} {"命令"="init", "数据"=variant} ("元素")) -> ()  [unwired: 2 in, 3 out]
              }
              frame Enabled {
              }
            }
            n186 = Wait (ms)(milliseconds to wait=u32 2000 ("等待时间（毫秒）")) -> ()  [unwired: 1 out]
          }
        }
        n187 = call <vilib>:"Clear Errors.vi"("error in (no error)"=w342) -> ("error out"=w341:errorcluster)  [unwired: 5 in, 1 out]
      }
    }
    n188 = Unbundle By Name(w196) -> ("status"=→"通讯故障":bool)
  }
  n189 = property on="多列列表框" class="MCListbox (严格)"("ItemNames"=string[][] [["待机"], ["初始化"], ["外部管路润洗"], ["内部管路润洗"], ["采样"], ["沉淀"], ["配水"], ["外部管路反冲洗"], ["内部管路反冲洗"], ["采样池储水"], ["结束"]] ("项名")) -> ()  [unwired: 2 in, 2 out]
  n190 = call-dynamic "Close Session.vi"("error in (no error)"=w2, "MB session in"=w1) -> ()  [unwired: 9 in, 1 out]
